vi "2019-05-14_Global_Variable.vi"() -> ()   [LabVIEW 2018]
uses:
  ex_Global.vi
panel:
  in  "정지 버튼":bool
  out "웨이브폼 차트":dbl(graph)
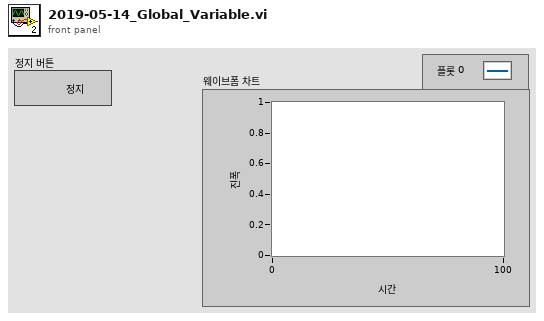
[diagram p1: front panel]
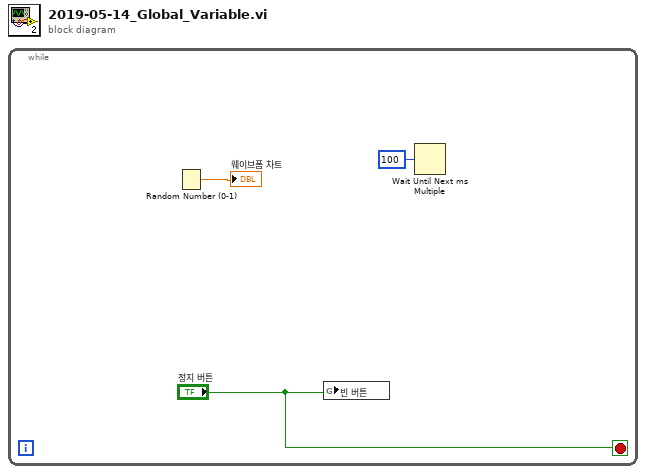
[diagram p0: block diagram]
diagram:
  n1 = while {
    stop <- "정지 버튼" stop-if-true
    n2 = Random Number (0-1)() -> (number: 0 to 1=→"웨이브폼 차트":dbl)
    n3 = global write "ex_Global.vi" "빈 버튼"("정지 버튼") -> ()
    n4 = Wait Until Next ms Multiple(millisecond multiple=u32 100 ("ms 배수")) -> ()  [unwired: 1 out]
  }
